vi "DMSV.subscribe_CS_services.vi"(0 "csServices":i32[][](array[numeric]), 1 "csNotifiers":refnum<notifier>[][](array[refnum]), 2 "csSystems":string[](array[string]), 5 "error in (no error)":errorcluster) -> (14 "csServices (out)":i32[][](array[numeric]), 15 "csNotifiers (out)":refnum<notifier>[][](array[refnum]), 19 "error out":errorcluster)   [LabVIEW 2014, in "DMSViewer.lvlib"]
doc: "Subscribes the domain viewer to DIM services providing information about CS systems.\n\nauthor: Dietrich Beck, GSI\n\nLicense Agreement for this software:\n\nCopyright (C)\nGesellschaft für Schwerionenforschung, GSI\nPlanckstr. 1\n64291 Darmstadt\nGermany\n\nContact: D.Beck@gsi.de \n\nThis program is free software; you can redistribute it and/or modify it under the terms of the GNU General Public License as published by the Free Software Foundation; either version 2 of the license, or (at your option) any later version.\n\nThis program is distributed in the hope that it will be useful, but WITHOUT ANY WARRANTY; without even the implied warranty of MERCHANTABILITY or FITNESS FOR A PARTICULAR PURPOSE. See the GNU General License for more details (http://www.gnu.org).\n\nGesellschaft für Schwerionenforschung, GSI\nPlanckstr. 1, 64291 Darmstadt, Germany\nFor all questions and ideas contact: M.Richter@gsi.de, H.Brand@gsi.de or D.Beck@gsi.de.\nLast update: 10-OCT-2004"
uses:
  DMSViewer.lvlib
  CSlibraries-extern/DimLVEvent/LVDimInterface/LVDimInterface.dim service type.ctl
  CSlibraries-extern/DimLVEvent/LVDimInterface/LVDimInterface.dic_info_service_notifier.vi
  CSlibraries-extern/DimLVEvent/LVDimInterface/LVDimInterface.lvlib
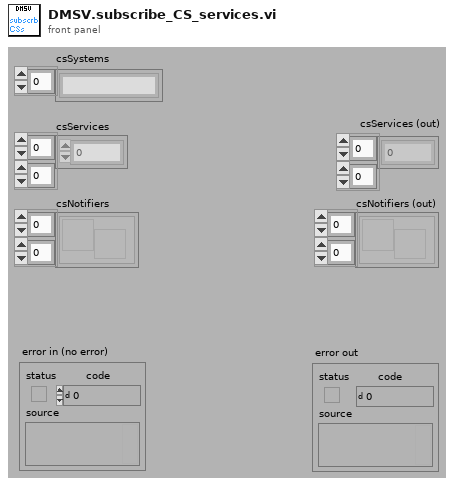
[diagram p1: front panel]
types:
  T1 = typedef "LVDimInterface.lvlib/LVDimInterface.dim service type.ctl" = u16
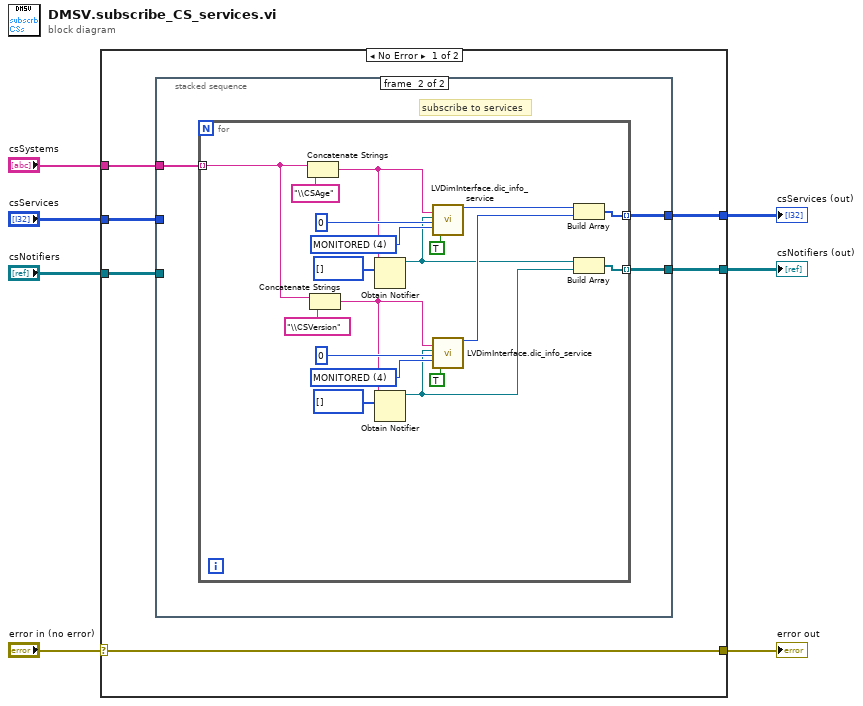
[diagram p0: block diagram]
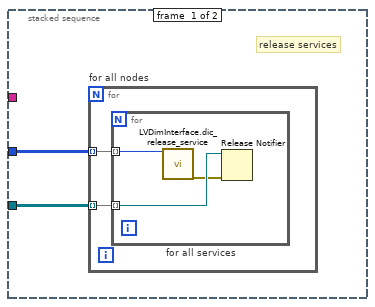
[diagram p2: hidden frame]
diagram:
  n1 = case shown="No Error" "error in (no error)" {
    selector: "error in (no error)" -> [w8 w45]
    tunnel: "csSystems" -> [w13 _]
    tunnel: [w8 w45] -> w5
    tunnel: [w12 w44] -> w4
    tunnel: [w11 w43] -> w3
    tunnel: "csServices" -> [w10 w44]
    tunnel: "csNotifiers" -> [w9 w43]
    frame No Error {
      n2 = stacked-sequence {
        tunnel: w13 -> [_ w23]
        tunnel: [_ w22] -> w12
        tunnel: [_ w21] -> w11
        tunnel: w10 -> [w15 _]
        tunnel: w9 -> [w14 _]
        frame #0 {
          # "release services"
          n3 = for "for all nodes" {
            tunnel: w15 -> [w17] mode=indexing
            tunnel: w14 -> [w16] mode=indexing
            n4 = for "for all services" {
              tunnel: w17 -> [w20] mode=indexing
              tunnel: w16 -> [w19] mode=indexing
              n5 = call "LVDimInterface.dic_release_service.vi"("callBackID"=w20) -> ("error out"=w18:errorcluster)  [unwired: 18 in]
              n6 = Release Notifier(notifier=w19, error in (no error)=w18) -> ()  [unwired: 1 in, 3 out]
            }
          }
        }
        frame #1 {
          # "subscribe to services"
          n7 = for {
            tunnel: w23 -> [w24] mode=indexing
            tunnel: [w26] -> w22 mode=indexing
            tunnel: [w25] -> w21 mode=indexing
            w34 = T1 4 items=["ONCE_ONLY"=1, "TIMED"=2, "MONITORED"=4] ("serviceType")
            w38 = T1 4 items=["ONCE_ONLY"=1, "TIMED"=2, "MONITORED"=4] ("serviceType")
            n8 = Concatenate Strings(w24, "\\CSAge" ("string")) -> (w36:string)
            n9 = Concatenate Strings(w24, "\\CSVersion" ("string")) -> (w31:string)
            n10 = Obtain Notifier(name (unnamed)=w36, notification data type=i8[] []) -> (notifier out=w28:refnum<notifier>)  [unwired: 2 in, 2 out]
            n11 = Obtain Notifier(name (unnamed)=w31, notification data type=i8[] []) -> (notifier out=w27:refnum<notifier>)  [unwired: 2 in, 2 out]
            n12 = call-poly "LVDimInterface.dic_info_service.vi"("serviceName"=w36, "notifierRef"=w28, "timeout [s]"=0, "serviceType"=w38, "stamped"=TRUE) -> ("callBackID"=w30:i32)  [unwired: 13 in, 1 out]
            n13 = call-poly "LVDimInterface.dic_info_service.vi"("serviceName"=w31, "notifierRef"=w27, "timeout [s]"=0, "serviceType"=w34, "stamped"=TRUE) -> ("callBackID"=w29:i32)  [unwired: 13 in, 1 out]
            n14 = Build Array(w30, w29) -> (w26:i32[])
            n15 = Build Array(w28, w27) -> (w25:refnum<notifier>[])
          }
        }
      }
    }
    frame Error {
    }
  }
  "error out" <- w5
  "csServices (out)" <- w4
  "csNotifiers (out)" <- w3
